vi "(Sub) to_HEX.vi"(1 "IN_10진수":dbl format="%#_f") -> (0 "OUT_16진수":string)   [LabVIEW 2017]
panel:
  out "*(type *) &x":string
  out "음수?":bool
  out "Numeric":u8
  out "*(타입 *) &x 2":string
  out "*(타입 *) &x":string
  out "숫자 2":u8 format="%02.0f"
  out "숫자":u8 format="%02.0f"
  out "소수점 3-4":string
  out "소수점 1-2":string
  out "소수":string
  out "정수":string
  out "10진수 문자열":string
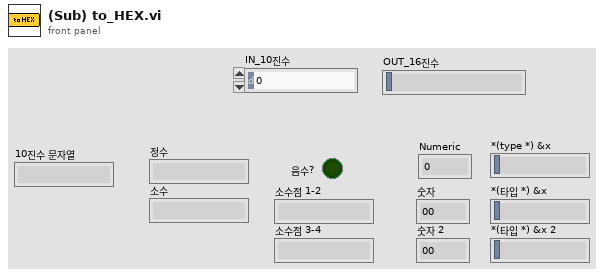
[diagram p1: front panel]
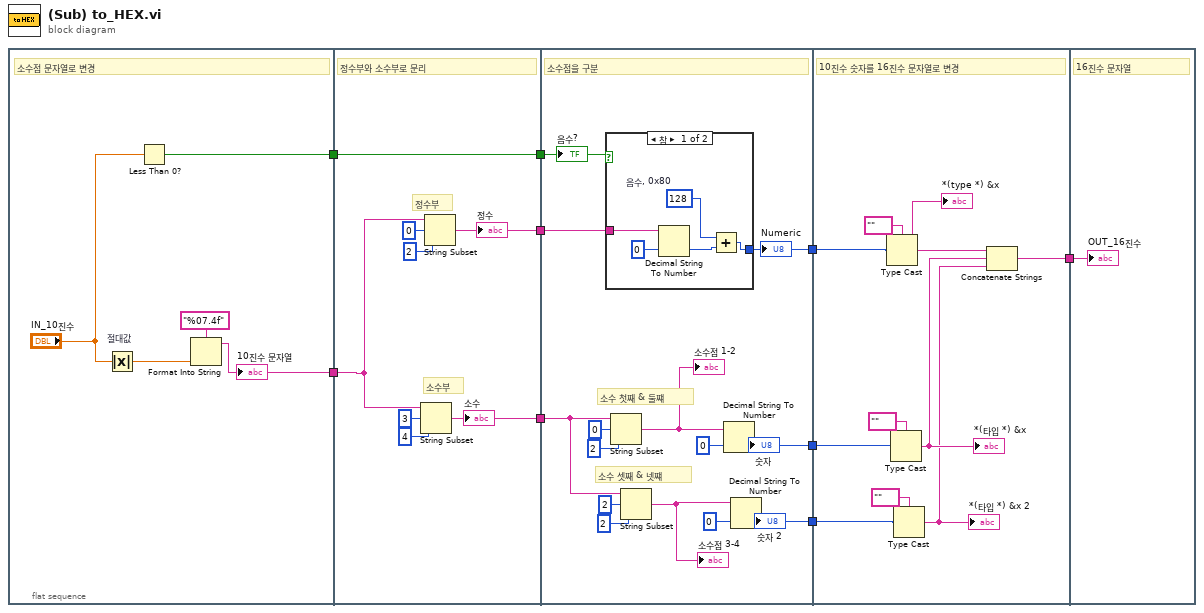
[diagram p0: block diagram]
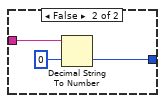
[diagram p2: hidden frame]
diagram:
  n1 = flat-sequence {
    tunnel: [w12] -> w3
    tunnel: [w13] -> w1
    tunnel: w3 -> [w21]
    tunnel: [w20] -> w9
    tunnel: [w19] -> w8
    tunnel: [w18] -> w2
    tunnel: w1 -> [w18]
    tunnel: w9 -> [w28]
    tunnel: w8 -> [w27]
    tunnel: [w26] -> w7
    tunnel: [w25] -> w6
    tunnel: [w23] -> w5
    tunnel: w2 -> [w24]
    tunnel: w7 -> [w51]
    tunnel: w6 -> [w50]
    tunnel: w5 -> [w45]
    tunnel: [w46] -> w4
    tunnel: w4 -> [w55]
    frame #0 {
      # "소수점 문자열로 변경"
      n2 = Absolute Value "절대값"(x="IN_10진수") -> (abs(x)=w11:dbl)
      n3 = Less Than 0?(x="IN_10진수") -> (x < 0?=w13:bool)
      n4 = Format Into String(format string="%07.4f", w11) -> (resulting string=w12:string)  [unwired: 2 in, 1 out]
      "10진수 문자열" <- w12
    }
    frame #1 {
      # "소수부"
      # "정수부"
      # "정수부와 소수부로 문리"
      n5 = String Subset(string=w21, offset (0)=3, length (rest)=4 ("length (rest)")) -> (substring=w20:string)
      "소수" <- w20
      n6 = String Subset(string=w21, offset (0)=0 ("오프셋(0)"), length (rest)=2 ("length (rest)")) -> (substring=w19:string)
      "정수" <- w19
    }
    frame #2 {
      # "소수 셋째 & 넷쨰"
      # "소수 첫째 & 둘쨰"
      # "소수점을 구분"
      n7 = case shown="참" w24 {
        tunnel: w27 -> [w40 w43]
        tunnel: [w38 w42] -> w23
        frame True {
          w37 = u8 128  # 음수, 0x80
          n8 = Decimal String To Number(string=w40, default (0L)=u8 0 ("기본(0 I32)")) -> (number=w39:u8)  [unwired: 1 in, 1 out]
          n9 = Add(x=w37, y=w39) -> (x+y=w38:u8)
        }
        frame False {
          n10 = Decimal String To Number(string=w43, default (0L)=u8 0 ("기본(0 I32)")) -> (number=w42:u8)  [unwired: 1 in, 1 out]
        }
      }
      "Numeric" <- w23
      n11 = String Subset(string=w28, offset (0)=0 ("오프셋(0)"), length (rest)=2 ("길이(나머지)")) -> (substring=w35:string)
      "소수점 1-2" <- w35
      n12 = String Subset(string=w28, offset (0)=2 ("오프셋(0)"), length (rest)=2 ("길이(나머지)")) -> (substring=w36:string)
      "소수점 3-4" <- w36
      n13 = Decimal String To Number(string=w35, default (0L)=u8 0 ("기본(0 I32)")) -> (number=w25:u8)  [unwired: 1 in, 1 out]
      "숫자" <- w25
      n14 = Decimal String To Number(string=w36, default (0L)=u8 0 ("기본(0 I32)")) -> (number=w26:u8)  [unwired: 1 in, 1 out]
      "숫자 2" <- w26
      "음수?" <- w24
    }
    frame #3 {
      # "10진수 숫자를 16진수 문자열로 변경"
      n15 = Type Cast(type="" ("CH No."), x=w45) -> (*(type *) &x=w49:string)
      "*(type *) &x" <- w49
      n16 = Type Cast(type="" ("CH No."), x=w50) -> (*(type *) &x=w48:string)
      "*(타입 *) &x" <- w48
      n17 = Type Cast(type="" ("CH No."), x=w51) -> (*(type *) &x=w47:string)
      "*(타입 *) &x 2" <- w47
      n18 = Concatenate Strings(w49, w48, w47) -> (w46:string)
    }
    frame #4 {
      # "16진수 문자열"
      "OUT_16진수" <- w55
    }
  }
